vi "Auto Intake Loop.vi"() -> (2 "Intake Power":dbl)   [LabVIEW 2016]
uses:
  Common Code/Intake Commands.ctl
  Robot Global Data.vi
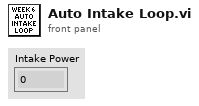
[diagram p1: front panel]
types:
  T1 = typedef "Intake Commands.ctl" = enum16{"Idle", "Intake", "Outtake"}
  T2 = typedef "Dashboard Packet.ctl" = cluster{"Intake Presets":T3}
  T3 = typedef "Intake Presets.ctl" = cluster{"Intake Power":dbl, "Outtake Power":dbl}
  T4 = typedef "Intake Command Cluster.ctl" = cluster{"Intake Mode":T5, "Intake Command":T1, "Intake Manual Power":dbl}
  T5 = typedef "Intake Mode.ctl" = enum16{"Manual", "Auto"}
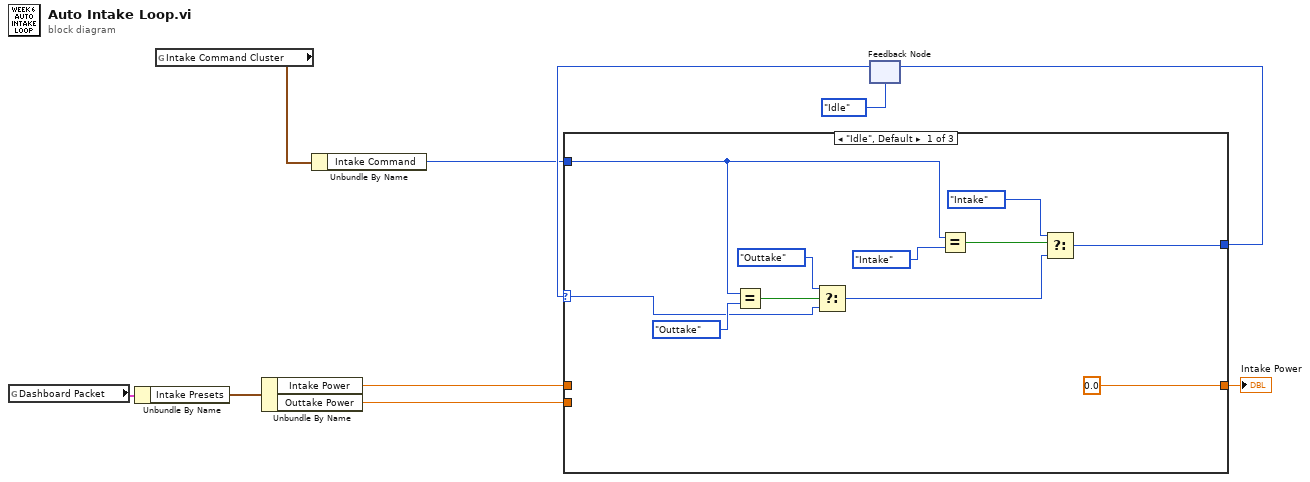
[diagram p0: block diagram]
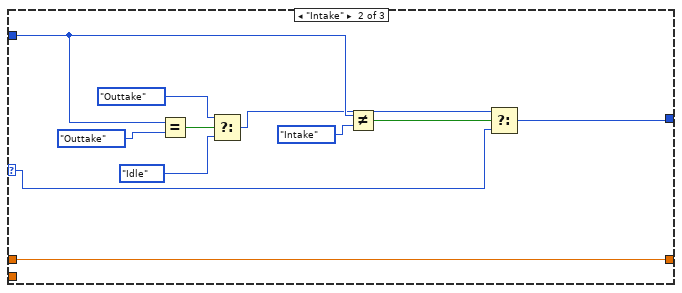
[diagram p2: hidden frame]
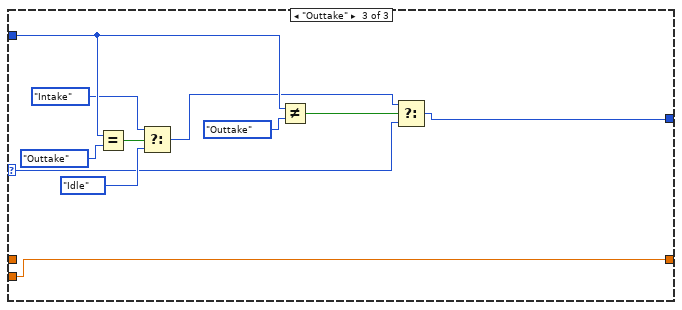
[diagram p3: hidden frame]
diagram:
  n1 = global read "Robot Global Data.vi" "Dashboard Packet"() -> (w4:T2)
  n2 = Unbundle By Name(w4) -> ("Intake Presets"=w3:T3)
  n3 = global read "Robot Global Data.vi" "Intake Command Cluster"() -> (w10:T4)
  n4 = Unbundle By Name(w3) -> ("Intake Power"=w2:dbl, "Outtake Power"=w1:dbl)
  n5 = Unbundle By Name(w10) -> ("Intake Command"=w7:T1)
  n6 = feedback #1(Intake_Commands."Idle" ("Intake Command")) -> (w8:T1)
  n7 = case shown="\"Idle\", Default" w8 {
    selector: w8 -> [w13 w23 w34]
    tunnel: [w18 w22 w33] -> w6
    tunnel: w7 -> [w16 w28 w38]
    tunnel: [0.0 w32 w43] -> w5
    tunnel: w2 -> [_ w32 _]
    tunnel: w1 -> [_ _ w43]
    frame "Idle", Default {
      n8 = Equal?(x=w16, y=Intake_Commands."Outtake" ("Intake Command")) -> (x = y?=w15:bool)
      n9 = Select(t=Intake_Commands."Outtake" ("Intake Command"), s=w15, f=w13) -> (s? t:f=w12:T1)
      n10 = Equal?(x=w16, y=Intake_Commands."Intake" ("Intake Command")) -> (x = y?=w21:bool)
      n11 = Select(t=Intake_Commands."Intake" ("Intake Command"), s=w21, f=w12) -> (s? t:f=w18:T1)
    }
    frame "Intake" {
      n12 = Equal?(x=w28, y=Intake_Commands."Outtake" ("Intake Command")) -> (x = y?=w27:bool)
      n13 = Select(t=Intake_Commands."Outtake" ("Intake Command"), s=w27, f=Intake_Commands."Idle" ("Intake Command")) -> (s? t:f=w24:T1)
      n14 = Not Equal?(x=w28, y=Intake_Commands."Intake" ("Intake Command")) -> (x != y?=w30:bool)
      n15 = Select(t=w24, s=w30, f=w23) -> (s? t:f=w22:T1)
    }
    frame "Outtake" {
      n16 = Equal?(x=w38, y=Intake_Commands."Outtake" ("Intake Command")) -> (x = y?=w39:bool)
      n17 = Select(t=Intake_Commands."Intake" ("Intake Command"), s=w39, f=Intake_Commands."Idle" ("Intake Command")) -> (s? t:f=w35:T1)
      n18 = Not Equal?(x=w38, y=Intake_Commands."Outtake" ("Intake Command")) -> (x != y?=w41:bool)
      n19 = Select(t=w35, s=w41, f=w34) -> (s? t:f=w33:T1)
    }
  }
  "Intake Power" <- w5
  n20 = feedback-in #1(w6) -> ()
